vi "Datasheet ASCII Channel Data.vi"(1 "Channel Data":T1[](array[typedef])) -> (0 "HTM Table Rows":string)   [LabVIEW 2011]
uses:
  TDMS/TDMS Channel (Sxx).ctl
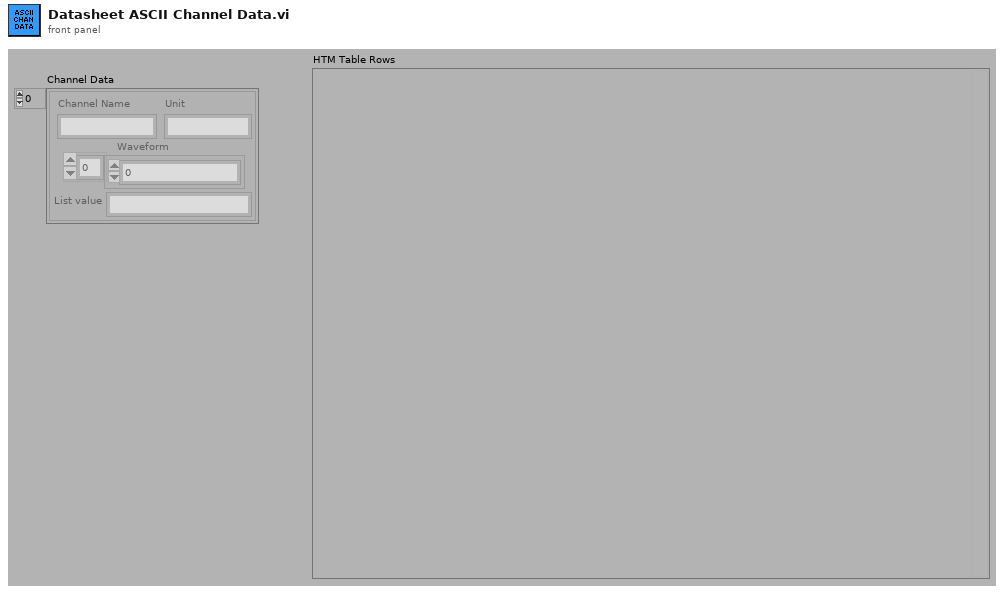
[diagram p1: front panel]
types:
  T1 = typedef "TDMS Channel (Sxx).ctl" = cluster{"Channel Name":string, "Waveform":dbl[], "Unit":string, "List value":string}
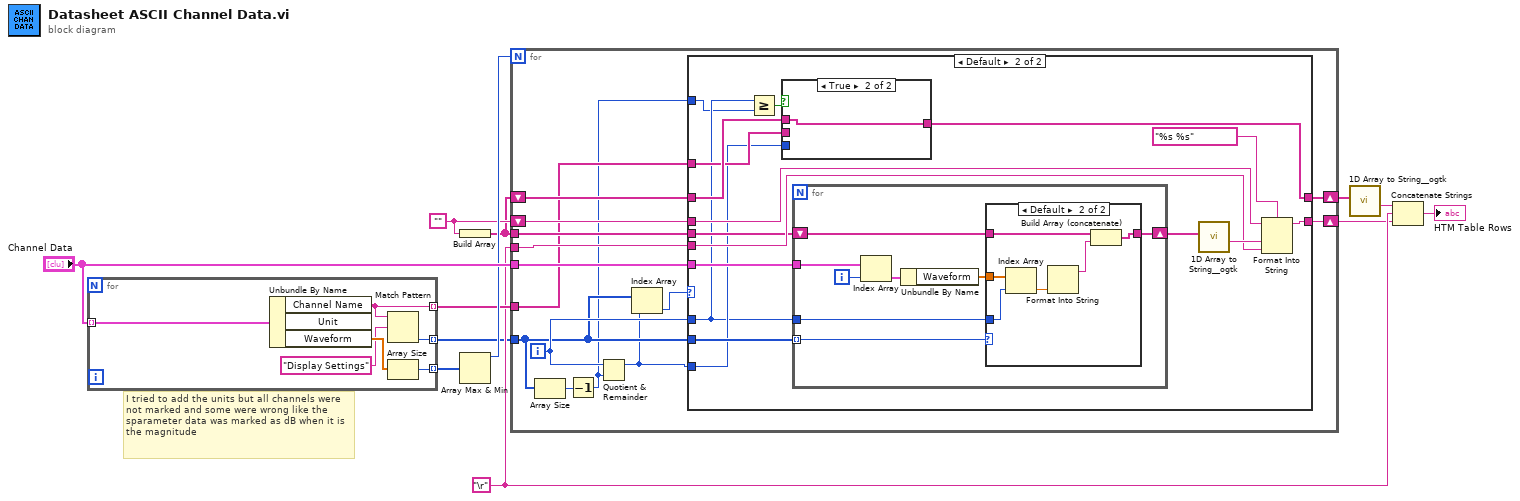
[diagram p0: block diagram]
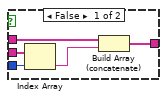
[diagram p3: hidden frame]
diagram:
  w8 = ""
  w6 = "\r" ("format string")
  # "I tried to add the units but all channels were not marked and some were wrong like the sparameter data was marked as dB when it is the magnitude"
  n1 = for {
    tunnel: "Channel Data" -> [w18] mode=indexing
    tunnel: [w14] -> w9 mode=indexing
    tunnel: [w16] -> w11 mode=indexing
    tunnel: [w13] -> w1 mode=indexing
    n2 = Unbundle By Name(w18) -> ("Channel Name"=w14:string, "Waveform"=w17:dbl[])  [unwired: 1 out]
    n3 = Match Pattern(string=w14, regular expression="Display Settings" ("string")) -> (offset past match=w13:i32)  [unwired: 1 in, 3 out]
    n4 = Array Size(array=w17) -> (size(s)=w16:i32)
  }
  n5 = Build Array(w8) -> (w2:string[])
  n6 = Array Max & Min(array=w11) -> (max value=w10:i32)  [unwired: 3 out]
  n7 = for {
    N: w10 -> [_]
    shift-right: [w31] -> w5
    shift-left: w8 -> [w29]
    tunnel: "Channel Data" -> [w32]
    tunnel: w6 -> [w30]
    tunnel: w9 -> [w24]
    shift-right: [w27] -> w7
    shift-left: w2 -> [w28]
    tunnel: w2 -> [w26]
    tunnel: w1 -> [w21]
    i -> [w25]
    n8 = Array Size(array=w21) -> (size(s)=w23:i32)
    n9 = Decrement(x=w23) -> (x-1=w19:i32)
    n10 = Quotient & Remainder(x=w25, y=w19) -> (x-y*floor(x/y)=w20:i32)  [unwired: 1 out]
    n11 = Index Array(array=w21, index=w20) -> (element=w22:i32)
    n12 = case shown="Default" w22 {
      tunnel: w32 -> [_ w50]
      tunnel: w25 -> [_ w36]
      tunnel: w29 -> [w34 w48]
      tunnel: [w34 w47] -> w31
      tunnel: w30 -> [_ w46]
      tunnel: w28 -> [w33 w44]
      tunnel: [w33 w43] -> w27
      tunnel: w26 -> [_ w42]
      tunnel: w21 -> [_ w41]
      tunnel: w24 -> [_ w39]
      tunnel: w20 -> [_ w37]
      tunnel: w19 -> [_ w35]
      frame 0.. {
      }
      frame Default {
        n13 = Greater Or Equal?(x=w36, y=w35) -> (x >= y?=w38:bool)
        n14 = case shown="True" w38 {
          tunnel: w44 -> [w55 w56]
          tunnel: [w54 w56] -> w43
          tunnel: w39 -> [w52 _]
          tunnel: w37 -> [w51 _]
          frame False {
            n15 = Index Array(array=w52, index=w51) -> (element=w53:string)
            n16 = Build Array (concatenate)(w55, w53) -> (w54:string[])
          }
          frame True {
          }
        }
        n17 = for {
          tunnel: w50 -> [w60]
          shift-right: [w61] -> w40
          shift-left: w42 -> [w63]
          tunnel: w41 -> [w62] mode=indexing
          tunnel: w36 -> [w58]
          i -> [w57]
          n18 = Index Array(array=w60, index=w57) -> (element=w59:T1)
          n19 = Unbundle By Name(w59) -> ("Waveform"=w64:dbl[])
          n20 = case shown="Default" w62 {
            tunnel: w64 -> [_ w71]
            tunnel: w63 -> [w65 w68]
            tunnel: [w65 w67] -> w61
            tunnel: w58 -> [_ w66]
            frame 0.. {
            }
            frame Default {
              n21 = Index Array(array=w71, index=w66) -> (element=w70:dbl)
              n22 = Format Into String(w70) -> (resulting string=w69:string)  [unwired: 3 in, 1 out]
              n23 = Build Array (concatenate)(w68, w69) -> (w67:string[])
            }
          }
        }
        n24 = call "1D Array to String__ogtk.vi"("Array of Strings"=w40) -> ("delimited string"=w49:string)  [unwired: 10 in]
        n25 = Format Into String(format string="%s %s", initial string=w48, w49, w46) -> (resulting string=w47:string)  [unwired: 1 in, 1 out]
      }
    }
  }
  n26 = call "1D Array to String__ogtk.vi"("Array of Strings"=w7) -> ("delimited string"=w3:string)  [unwired: 10 in]
  n27 = Concatenate Strings(w3, w6, w5) -> (→"HTM Table Rows":string)
